vi "Charger_Set Status Color.vi"(0 "error in":errorcluster, 4 "Status Refnum":T1) -> (7 "error out":errorcluster)   [LabVIEW 2020]
uses:
  Charger_Status Refnum.ctl
  Drivers/Charger Test Set/Charger_Input Control.ctl
panel:
  out "status string":string
  in  "Labels":string[](array[string])=["More than one IPG found", "IPG charging error", "error", "Ready to load", "Searching for IPG", "Found IPG", "No IPG Found", "Opening Telemetry session", "Telemetry session open", "Failed to establish Telemetry session", "Terminated by user", "Charging in progress", "IPG charge completed ", "VBAT >=", "<<default>>"]
  in  "BG":u32[](array[colorbox])=[16711680, 16711680, 16711680, 13816530, 8454143, 16777224, 16635906, 32960, 32960, 16744512, 16635906, 32960, 6618880, 32768, 16448250]
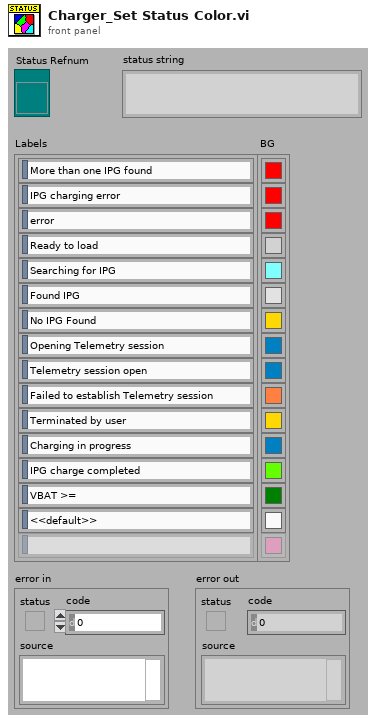
[diagram p1: front panel]
types:
  T1 = typedef "Charger_Status Refnum.ctl" = refnum<vi>
  T2 = typedef "Charger_Input Control.ctl" = cluster{"address":refnum<visa-resource-name>, "position":i32, "setpoint":dbl}
  T3 = cluster{"MICS ID":u32, "VBAT":dbl, "ChargingState":string, "VBAT Slide":dbl, "Status":string, "TemperatureLevel":dbl, "IPG_ReceivedLevel":dbl, "VBAT Target":dbl, "Charger Setpoint":dbl, "Index":i32, "Ready":bool, "Charger Inputs":T2, "MICS Inputs":cluster{"address":refnum<visa-resource-name>, "chan":u16, "ID":u32}}
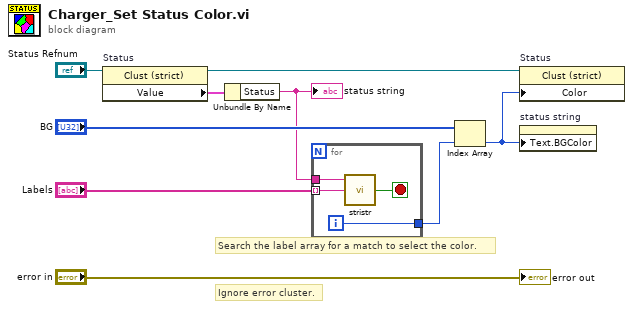
[diagram p0: block diagram]
diagram:
  # "Ignore error cluster."
  # "Search the label array for a match to select the color."
  n1 = property on="Status" class="Clust (strict)"(reference="Status Refnum") -> (reference out=w9:T1, "Value"=w2:T3)  [unwired: 1 in, 1 out]
  n2 = Unbundle By Name(w2) -> ("Status"=w1:string)
  "status string" <- w1
  n3 = for {
    tunnel: [w13] -> w3
    tunnel: "Labels" -> [w11] mode=indexing
    tunnel: w1 -> [w12]
    i -> [w13]
    stop <- w10 stop-if-true
    n4 = call "stristr.vi"("Substring"=w11, "Input String"=w12) -> ("found"=w10:bool)  [unwired: 1 in, 2 out]
  }
  n5 = Index Array(array="BG", index=w3) -> (element=w4:u32)
  n6 = property on="Status" class="Clust (strict)"(reference=w9, "Color"=w4) -> ()  [unwired: 1 in, 2 out]
  n7 = property on="status string" class="Str"("Text.BGColor"=w4) -> ()  [unwired: 2 in, 2 out]
  "error out" <- "error in"
